vi "FRCts20_Backend_Test_Team_GET.vi"(8 "error in (no error)":errorcluster, 11 "Team Index":u32) -> (0 "error out":errorcluster, 1 "Time (ms)":u32, 2 "Status":string, 3 "Team Out":T1, 5 "Success":bool)   [LabVIEW 2014, in "FRCts20_Backend_TestCode.lvlib"]
uses:
  FRCts20_Backend_TestCode.lvlib
  FRCts20_Backend_API/FRCts20_Backend_API_Team.ctl
  FRCts20_Backend_API/FRCts20_Backend_API_SW.ctl
  FRCts20_Backend_API/FRCts20_Backend_API_Status.ctl
  FRCts20_Backend_API/FRCts20_Backend_API_Command_Team.ctl
  FRCts20_Backend_API/FRCts20_Backend_API_Team.vi
  FRCts20_Backend_API/FRCts20_Backend_API.lvlib
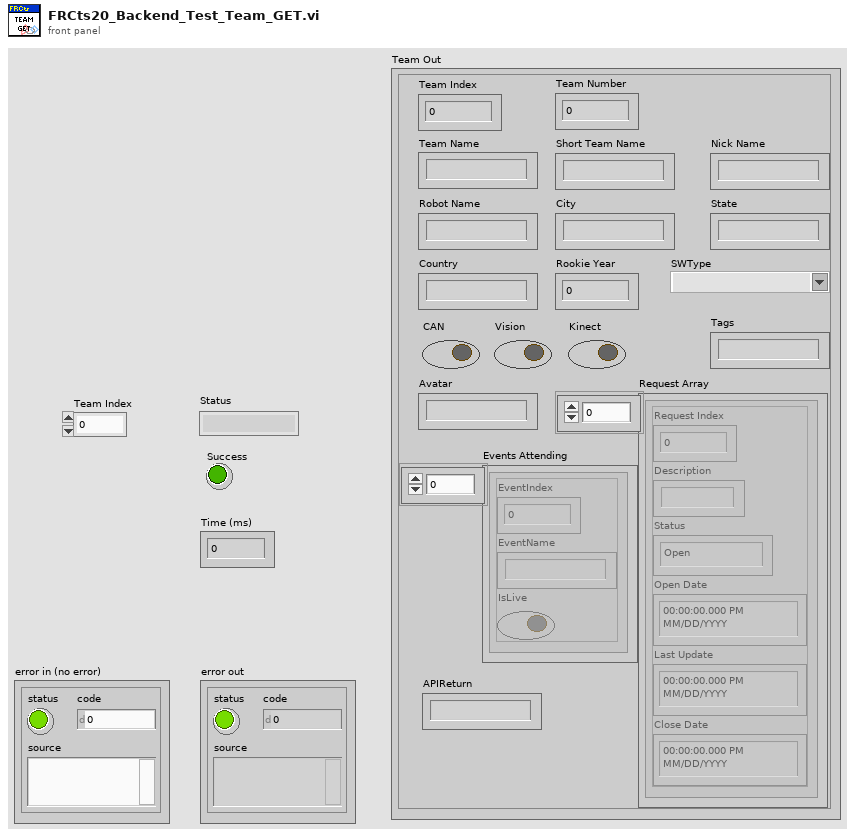
[diagram p1: front panel]
types:
  T1 = typedef "FRCts20_Backend_API.lvlib/FRCts20_Backend_API_Team.ctl" = cluster{"Team Index":u32, "Team Number":u32, "Team Name":string, "Short Team Name":string, "Nick Name":string, "Robot Name":string, "City":string, "State":string, "Country":string, "Rookie Year":u32, "SWType":T2, "CAN":bool, "Vision":bool, "Kinect":bool, "Tags":string, "Avatar":string, "Request Array":cluster{"Request Index":u32, "Description":string, "Status":T3, "Open Date":timestamp, "Last Update":timestamp, "Close Date":timestamp}[], "Events Attending":cluster{"EventIndex":dbl, "EventName":string, "IsLive":bool}[], "APIReturn":string}
  T2 = typedef "FRCts20_Backend_API.lvlib/FRCts20_Backend_API_SW.ctl" = string
  T3 = typedef "FRCts20_Backend_API.lvlib/FRCts20_Backend_API_Status.ctl" = enum16{"Open", "In Work", "Closed"}
  T4 = typedef "FRCts20_Backend_API.lvlib/FRCts20_Backend_API_Command_Team.ctl" = string
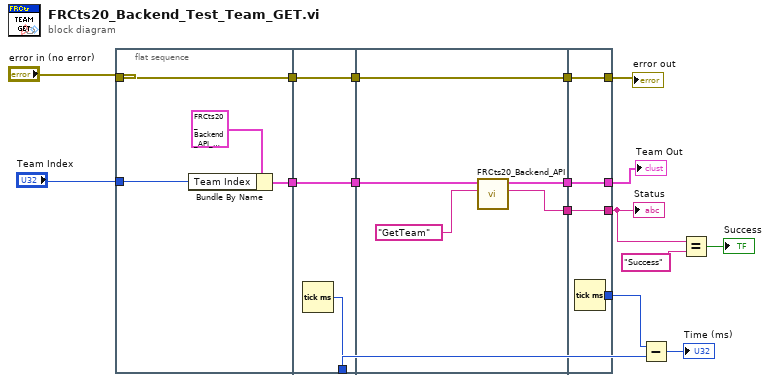
[diagram p0: block diagram]
diagram:
  n1 = flat-sequence {
    tunnel: "error in (no error)" -> [w21]
    tunnel: [w21] -> w17
    tunnel: [w19] -> w4
    tunnel: "Team Index" -> [w18]
    tunnel: [w24] -> w7
    tunnel: [w23] -> w16
    tunnel: w17 -> [w23]
    tunnel: w4 -> [w22]
    tunnel: [w22] -> w3
    tunnel: [w29] -> w15
    tunnel: w16 -> [w29]
    tunnel: [w28] -> w14
    tunnel: [w27] -> w5
    tunnel: w3 -> [w26]
    tunnel: [w33] -> w8
    tunnel: [w32] -> w10
    tunnel: w15 -> [w32]
    tunnel: [w31] -> w6
    tunnel: w14 -> [w31]
    tunnel: [w30] -> w2
    tunnel: w5 -> [w30]
    frame #0 {
      n2 = Bundle By Name(cluster=T1 {"Team Index"=0, "Team Number"=0, "Team Name"="", "Short Team Name"="", "Nick Name"="", "Robot Name"="", "City"="", "State"="", "Country"="", "Rookie Year"=0, "SWType"="", "CAN"=FALSE, "Vision"=FALSE, "Kinect"=FALSE, "Tags"="", "Avatar"="", "Request Array"=[], "Events Attending"=[], "APIReturn"=""} ("Team In"), "Team Index"=w18) -> (w19:T1)
    }
    frame #1 {
      n3 = Tick Count (ms)() -> (millisecond timer value=w24:u32)
    }
    frame #2 {
      n4 = call-poly "FRCts20_Backend_API.vi"("Command"=T4 "GetTeam", "Team In"=w26) -> ("Status"=w28:string, "Team Out"=w27:T1)  [unwired: 7 in, 1 out]
    }
    frame #3 {
      n5 = Tick Count (ms)() -> (millisecond timer value=w33:u32)
    }
  }
  n6 = Subtract(x=w8, y=w7) -> (x-y=→"Time (ms)":u32)
  n7 = Equal?(x=w6, y="Success") -> (x = y?=→"Success":bool)
  "Status" <- w6
  "error out" <- w10
  "Team Out" <- w2
